vi "GetTorqueInRange.vi"(9 "Motor Characteristics":T1, 10 "Pod Configuration":T2, 11 "Torque":dbl) -> (3 "In Range":bool)   [LabVIEW 2014]
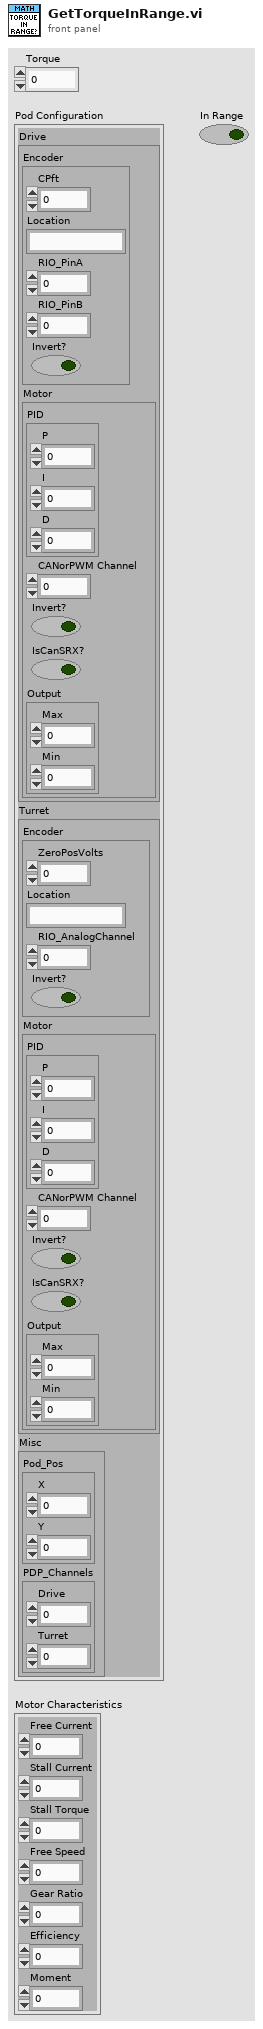
[diagram p1: front panel]
types:
  T1 = cluster{"Free Current":dbl, "Stall Current":dbl, "Stall Torque":dbl, "Free Speed":dbl, "Gear Ratio":dbl, "Efficiency":dbl, "Moment":dbl}
  T2 = cluster{"Drive":cluster{"Encoder":cluster{"CPft":dbl, "Location":string, "RIO_PinA":i32, "RIO_PinB":i32, "Invert?":bool}, "Motor":cluster{"PID":cluster{"P":dbl, "I":dbl, "D":dbl}, "CANorPWM Channel":i32, "Invert?":bool, "IsCanSRX?":bool, "Output":cluster{"Max":dbl, "Min":dbl}}}, "Turret":cluster{"Encoder":cluster{"ZeroPosVolts":dbl, "Location":string, "RIO_AnalogChannel":i32, "Invert?":bool}, "Motor":cluster{"PID":cluster{"P":dbl, "I":dbl, "D":dbl}, "CANorPWM Channel":i32, "Invert?":bool, "IsCanSRX?":bool, "Output":cluster{"Max":dbl, "Min":dbl}}}, "Misc":cluster{"Pod_Pos":cluster{"X":dbl, "Y":dbl}, "PDP_Channels":cluster{"Drive":i32, "Turret":i32}}}
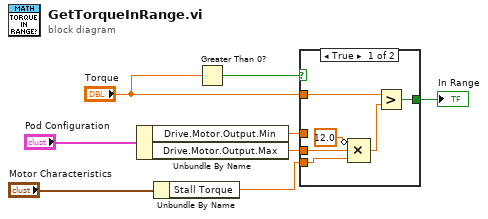
[diagram p0: block diagram]
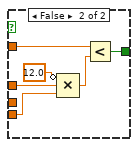
[diagram p2: hidden frame]
diagram:
  n1 = Unbundle By Name("Pod Configuration") -> ("Drive.Motor.Output.Min"=w1:dbl, "Drive.Motor.Output.Max"=w2:dbl)
  n2 = Unbundle By Name("Motor Characteristics") -> ("Stall Torque"=w7:dbl)
  n3 = Greater Than 0?(x="Torque") -> (x > 0?=w5:bool)
  n4 = case shown="True" w5 {
    tunnel: "Torque" -> [w11 w17]
    tunnel: [w14 w20] -> w8
    tunnel: w7 -> [w13 w19]
    tunnel: w2 -> [w9 _]
    tunnel: w1 -> [_ w15]
    frame True {
      n5 = Compound Arithmetic op=MULTIPLY(invert 12.0 ("value"), w9, w13) -> (w10:dbl)
      n6 = Greater?(x=w11, y=w10) -> (0:w14:bool)
    }
    frame False {
      n7 = Compound Arithmetic op=MULTIPLY(invert 12.0 ("value"), w15, w19) -> (w16:dbl)
      n8 = Less?(x=w17, y=w16) -> (x < y?=w20:bool)
    }
  }
  "In Range" <- w8
